vi "plot states.vi"(6 "Units":string(combo), 8 "Economizer?":bool, 9 "Power":dbl, 10 "fluid name":u16(ring)=17 items=["AIR.MIX", "AMARILLO.MIX", "EKOFISK.MIX", "GLFCOAST.MIX", "HIGHCO2.MIX", "HIGHN2.MIX", "NGSAMPLE.MIX", "R401A.MIX", "R401B.MIX", "R401C.MIX", "R402A.MIX", "R402B.MIX", "R403A.MIX", "R403B.MIX", "R405A.MIX", "R406A.MIX", "R407A.MIX", "R407B.MIX", "R407C.MIX", "R407D.MIX", "R407E.MIX", "R408A.MIX", "R409A.MIX", "R409B.MIX", "R410A.PPF", "R410B.MIX", "R411A.MIX", "R411B.MIX", "R412A.MIX", "R413A.MIX", "R414B.MIX", "R415A.MIX", "R415B.MIX", "R416A.MIX", "R417A.MIX", "R417B.MIX", "R417C.MIX", "R418A.MIX", "R419A.MIX", "R419B.MIX", "R420A.MIX", "R421A.MIX", "R421B.MIX", "R422A.MIX", "R422B.MIX", "R422C.MIX", "R422D.MIX", "R423A.MIX", "R424A.MIX", "R425A.MIX", "R426A.MIX", "R427A.MIX", "R428A.MIX", "R429A.MIX", "R430A.MIX", "R431A.MIX", "R432A.MIX", "R433A.MIX", "R433B.MIX", "R433C.MIX", "R434A.MIX", "R435A.MIX", "R436A.MIX", "R436B.MIX", "R437A.MIX", "R438A.MIX", "R439A.MIX", "R440A.MIX", "R441A.MIX", "R442A.MIX", "R443A.MIX", "R444A.MIX", "R444B.MIX", "R445A.MIX", "R446A.MIX", "R447A.MIX", "R448A.MIX", "R449A.MIX", "R449B.MIX", "R450A.MIX", "R451A.MIX", "R451B.MIX", "R452A.MIX", "R452B.MIX", "R452C.MIX", "R453A.MIX", "R454A.MIX", "R454B.MIX", "R454C.MIX", "R455A.MIX", "R456A.MIX", "R457A.MIX", "R459A.MIX", "R459B.MIX", "R460A.MIX", "R460B.MIX", "R500.MIX", "R501.MIX", "R502.MIX", "R503.MIX", "R504.MIX", "R507A.MIX", "R508A.MIX", "R508B.MIX", "R509A.MIX", "R510A.MIX", "R511A.MIX", "R512A.MIX", "R513A.MIX", "R513B.MIX", "R515A.MIX", "ammonia.fld", "butane.fld", "ethane.fld", "propane.fld", "R11.fld", "R113.fld", "R114.fld", "R115.fld", "R116.fld", "R12.fld", "R123.fld", "R124.fld", "R125.fld", "R13.fld", "R134a.fld", "R14.fld", "R141b.fld", "R142b.fld", "R143a.fld", "R152a.fld", "R161.fld", "R21.fld", "R218.fld", "R22.fld", "R227ea.fld", "R23.fld", "R236ea.fld", "R236fa.fld", "R245ca.fld", "R245fa.fld", "R32.fld", "R41.fld", "R1216.fld", "RC318.fld", "water.fld", "1butene.fld", "acetone.fld", "argon.fld", "benzene.fld", "c1cc6.fld", "c2butene.fld", "c3cc6.fld", "c4f10.fld", "c5f12.fld", "c11.fld", "c12.fld", "cf3i.fld", "CO.fld", "CO2.fld", "COS.fld", "cyclohex.fld", "cyclopen.fld", "cyclopro.fld", "D2.fld", "D2O.fld", "D4.fld", "D5.fld", "D6.fld", "decane.fld", "dee.fld", "dmc.fld", "dme.fld", "ebenzene.fld", "ethanol.fld", "ethylene.fld", "flourine.fld", "H2S.fld", "HCl.fld", "helium.fld", "heptane.fld", "hexane.fld", "hydrogen.fld", "ibutene.fld", "ihexane.fld", "ioctane.fld", "ipentane.fld", "isobutan.fld", "krypton.fld", "MD2M.fld", "MD3M.fld", "MD4M.fld", "MDM.fld", "methane.fld", "methanol.fld", "mlinolea.fld", "mlinolen.fld", "MM.fld", "moleate.fld", "mpalmita.fld", "mstearat.fld", "mxylene.fld", "N2O.fld", "neon.fld", "neopentn.fld", "NF3.fld", "nitrogen.fld", "nonane.fld", "novec649.fld", "octane.fld", "orthohyd.fld", "oxygen.fld", "parahyd.fld", "pentane.fld", "propylen.fld", "propyne.fld", "pxylene.fld", "R365MFC.fld", "R1233zd.fld", "R1234yf.fld", "R1234ze.fld", "RE143a.fld", "RE245cb2.fld", "RE245fa2.fld", "RE347mcc.fld", "sf6.fld", "SO2.fld", "T2butene.fld", "xenon.fld"], 11 "Data Cluster":T1) -> (0 "Ts output":cluster{dbl[], dbl[]}, 3 "ph output":cluster{dbl[], dbl[]})   [LabVIEW 2017]
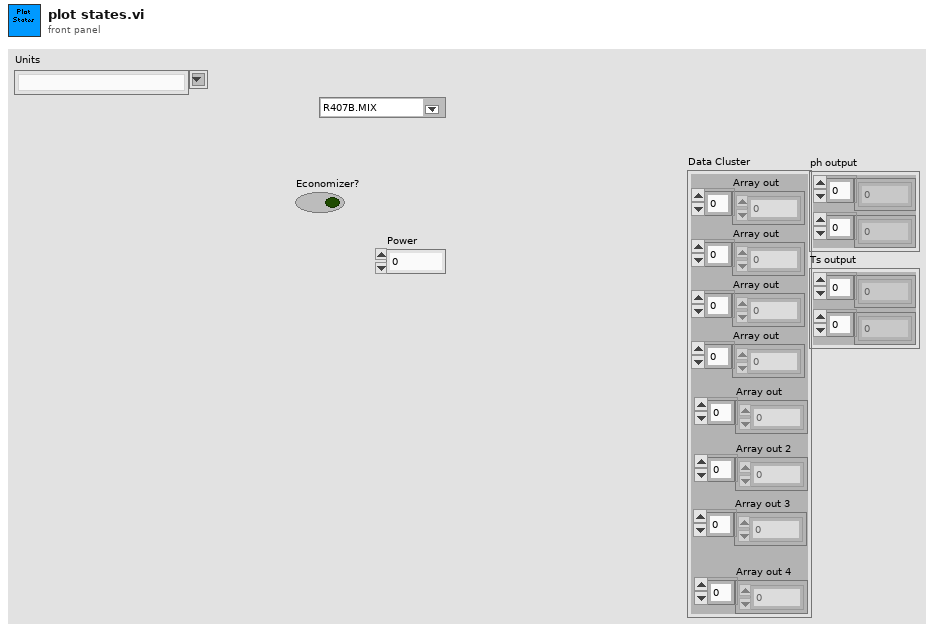
[diagram p1: front panel]
types:
  T1 = cluster{"Array out":dbl[], "Array out":dbl[], "Array out":dbl[], "Array out":dbl[], "Array out":dbl[], "Array out 2":dbl[], "Array out 3":dbl[], "Array out 4":dbl[]}
  T2 = enum16{"0", "PS", "HS", "T", "P", "TP", "TH", "TS", "PH", "PQ", "TQ"}
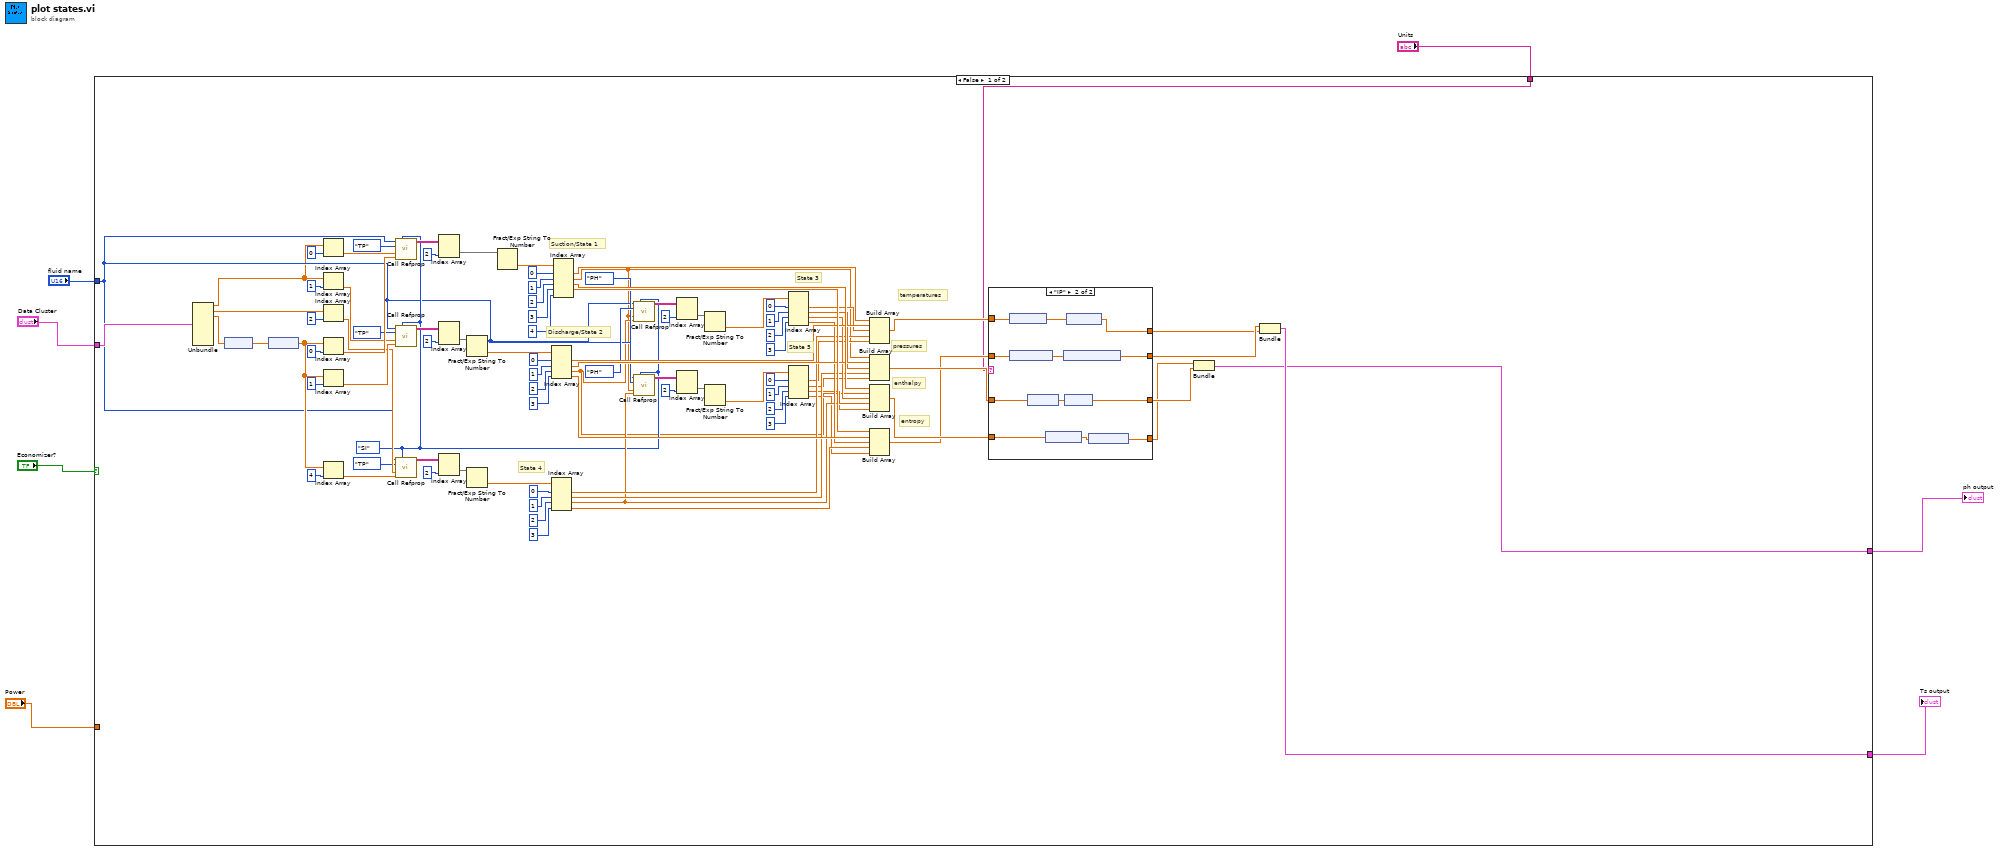
[diagram p0: block diagram]
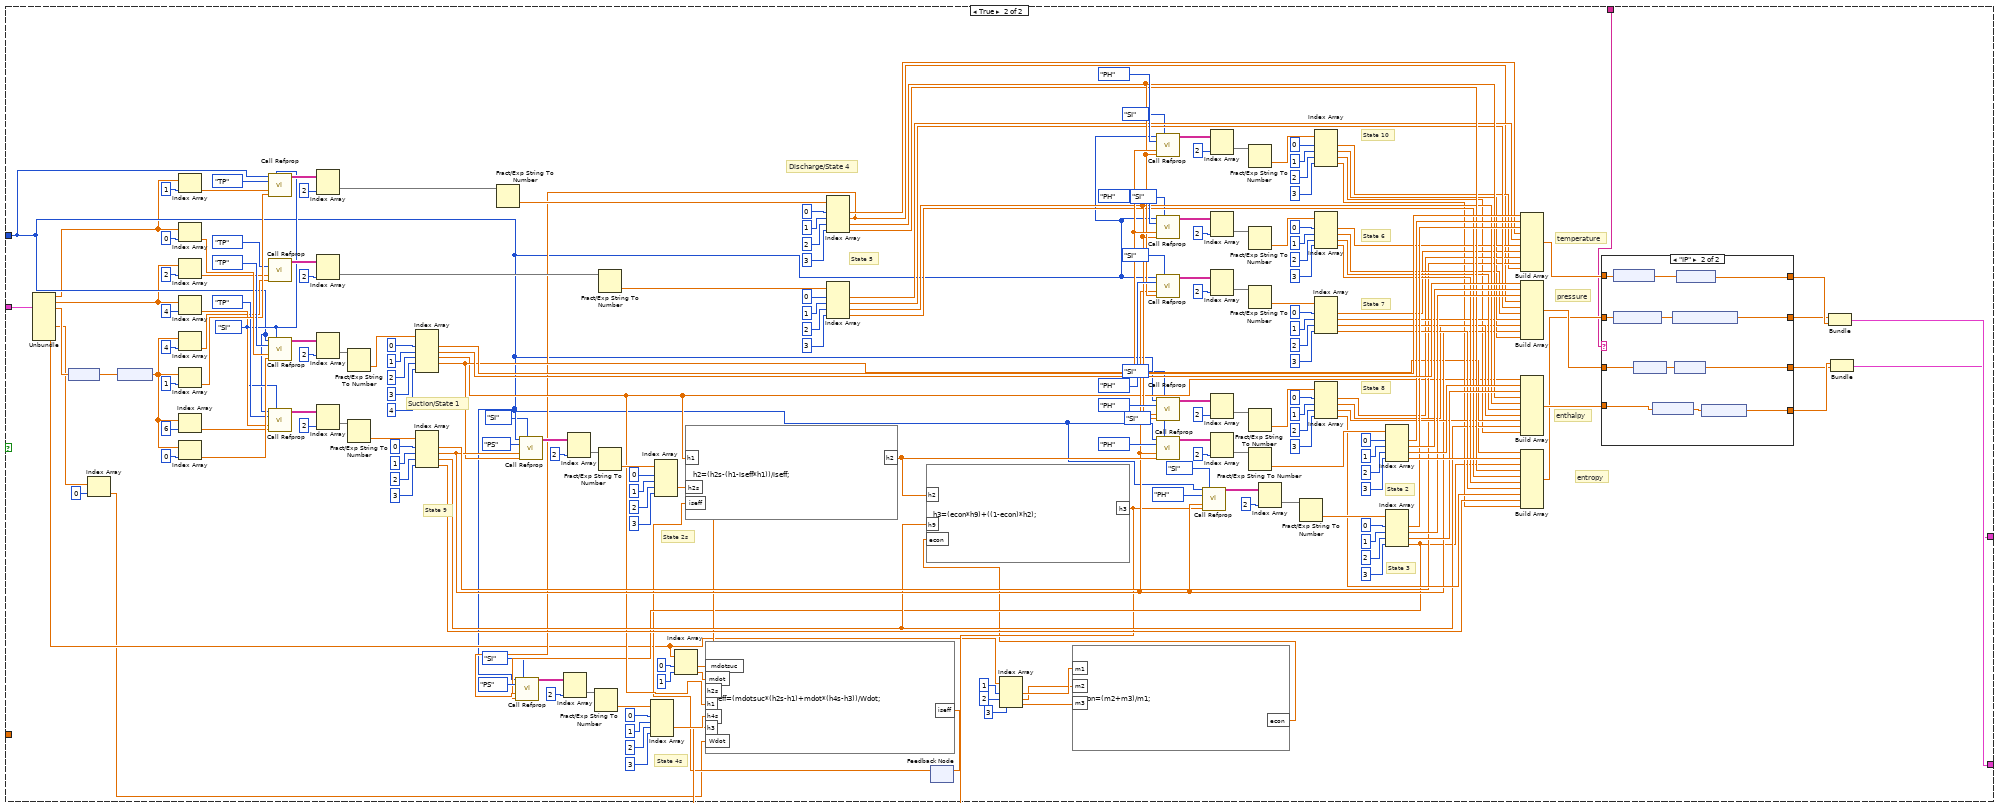
[diagram p3: hidden frame]
diagram:
  n1 = case shown="False" "Economizer?" {
    tunnel: [w24 w167] -> w6
    tunnel: [w23 w166] -> w5
    tunnel: "Data Cluster" -> [w22 w304]
    tunnel: "fluid name" -> [w21 w135]
    tunnel: "Power" -> [_ _]
    tunnel: "Units" -> [w10 w121]
    frame False {
      w25 = enum16{"SI", "IP"}."SI" ("units")
      # "State 5"
      # "State 4"
      # "State 3"
      # "Discharge/State 2"
      # "Suction/State 1"
      # "entropy"
      # "temperatures"
      # "enthalpy"
      # "pressures"
      n2 = Unbundle(w22) -> ("Array out"=w20:dbl[], "Array out"=w19:dbl[], "Array out"=w89:dbl[])  [unwired: 5 out]
      n3 = node(w89) -> (w90:dbl[unit][])
      n4 = node(w90) -> (w40:dbl[])
      n5 = Index Array(array=w20, index=0) -> (element=w101:dbl)
      n6 = Index Array(array=w20, index=1) -> (element=w83:dbl)
      n7 = Index Array(array=w19, index=2) -> (element=w54:dbl)
      n8 = Index Array(array=w40, index=0) -> (element=w100:dbl)
      n9 = Index Array(array=w40, index=1) -> (element=w82:dbl)
      n10 = Index Array(array=w40, index=4) -> (element=w53:dbl)
      n11 = call "Call Refprop.vi"("fluid name"=w21, "units"=w25, "InpCode"=T2."TP", "output_1"=w101, "output_2"=w100) -> ("data"=w99:string[][])  [unwired: 6 in, 4 out]
      n12 = call "Call Refprop.vi"("fluid name"=w21, "units"=w25, "InpCode"=T2."TP", "output_1"=w83, "output_2"=w82) -> ("data"=w81:string[][])  [unwired: 6 in, 4 out]
      n13 = call "Call Refprop.vi"("fluid name"=w21, "units"=w25, "InpCode"=T2."TP", "output_1"=w54, "output_2"=w53) -> ("data"=w52:string[][])  [unwired: 6 in, 4 out]
      n14 = Index Array(array=w99, index (col)=2 ("disabled index (col)")) -> (element=w97:string[])  [unwired: 1 in]
      n15 = Index Array(array=w81, index (col)=2 ("disabled index (col)")) -> (element=w79:string[])  [unwired: 1 in]
      n16 = Index Array(array=w52, index (col)=2 ("disabled index (col)")) -> (element=w50:string[])  [unwired: 1 in]
      n17 = Fract/Exp String To Number(string=w79) -> (number=w78:dbl[])  [unwired: 3 in, 1 out]
      n18 = Fract/Exp String To Number(string=w50) -> (number=w49:dbl[])  [unwired: 3 in, 1 out]
      n19 = Fract/Exp String To Number(string=w97) -> (number=w96:dbl[])  [unwired: 3 in, 1 out]
      n20 = Index Array(array=w78, index #1=0 ("index"), index #2=1 ("index"), index #3=2 ("index"), index #4=3 ("index")) -> (element #1=w72:dbl, element #2=w71:dbl, element #3=w9:dbl, element #4=w70:dbl)
      n21 = Index Array(array=w49, index #1=0 ("index"), index #2=1 ("index"), index #3=2 ("index"), index #4=3 ("index")) -> (element #1=w43:dbl, element #2=w42:dbl, element #3=w30:dbl, element #4=w41:dbl)
      n22 = Index Array(array=w96, index #1=0 ("index"), index #2=1 ("index"), index #3=2 ("index"), index #4=3 ("index"), index #5=4 ("index")) -> (element #1=w87:dbl, element #2=w8:dbl, element #3=w88:dbl, element #4=w86:dbl)  [unwired: 1 out]
      n23 = call "Call Refprop.vi"("fluid name"=w21, "units"=w25, "InpCode"=T2."PH", "output_1"=w8, "output_2"=w9) -> ("data"=w69:string[][])  [unwired: 6 in, 4 out]
      n24 = call "Call Refprop.vi"("fluid name"=w21, "units"=w25, "InpCode"=T2."PH", "output_1"=w8, "output_2"=w30) -> ("data"=w39:string[][])  [unwired: 6 in, 4 out]
      n25 = Index Array(array=w69, index (col)=2 ("disabled index (col)")) -> (element=w67:string[])  [unwired: 1 in]
      n26 = Index Array(array=w39, index (col)=2 ("disabled index (col)")) -> (element=w37:string[])  [unwired: 1 in]
      n27 = Fract/Exp String To Number(string=w67) -> (number=w66:dbl[])  [unwired: 3 in, 1 out]
      n28 = Fract/Exp String To Number(string=w37) -> (number=w36:dbl[])  [unwired: 3 in, 1 out]
      n29 = Index Array(array=w66, index #1=0 ("index"), index #2=1 ("index"), index #3=2 ("index"), index #4=3 ("index")) -> (element #1=w60:dbl, element #2=w59:dbl, element #3=w58:dbl, element #4=w57:dbl)
      n30 = Index Array(array=w36, index #1=0 ("index"), index #2=1 ("index"), index #3=2 ("index"), index #4=3 ("index")) -> (element #1=w29:dbl, element #2=w28:dbl, element #3=w27:dbl, element #4=w26:dbl)
      n31 = Build Array(w87, w72, w60, w43, w29) -> (w15:dbl[])
      n32 = Build Array(w8, w71, w59, w42, w28) -> (w18:dbl[])
      n33 = Build Array(w88, w9, w58, w30, w27) -> (w17:dbl[])
      n34 = Build Array(w86, w70, w57, w41, w26) -> (w16:dbl[])
      n35 = case shown="\"IP\"" w10 {
        tunnel: w18 -> [w107 w116]
        tunnel: w17 -> [w108 w115]
        tunnel: w16 -> [w106 w114]
        tunnel: w15 -> [w105 w113]
        tunnel: [w106 w112] -> w14
        tunnel: [w105 w111] -> w13
        tunnel: [w107 w110] -> w12
        tunnel: [w108 w109] -> w11
        frame "SI", Default {
        }
        frame "IP" {
          n36 = node(w113) -> (w118:dbl[unit][])
          n37 = node(w114) -> (w117:dbl[unit][])
          n38 = node(w116) -> (w119:dbl[unit][])
          n39 = node(w115) -> (w120:dbl[unit][])
          n40 = node(w117) -> (w112:dbl[])
          n41 = node(w119) -> (w110:dbl[])
          n42 = node(w118) -> (w111:dbl[])
          n43 = node(w120) -> (w109:dbl[])
        }
      }
      n44 = Bundle(w11, w12) -> (w23:cluster{dbl[], dbl[]})  [unwired: 1 in]
      n45 = Bundle(w14, w13) -> (w24:cluster{dbl[], dbl[]})  [unwired: 1 in]
    }
    frame True {
      w165 = enum16{"SI", "IP"}."SI" ("units")
      # "State 4s"
      # "entropy"
      # "temperature"
      # "enthalpy"
      # "pressure"
      # "State 2"
      # "State 10"
      # "State 8"
      # "State 7"
      # "State 6"
      # "State 5"
      # "State 2s"
      # "State 3"
      # "State 9"
      # "Discharge/State 4"
      # "Suction/State 1"
      n46 = Unbundle(w304) -> ("Array out"=w123:dbl[], "Array out"=w122:dbl[], "Array out"=w318:dbl[], "Array out"=w139:dbl[], "Array out 2"=w126:dbl[])  [unwired: 3 out]
      n47 = node(w318) -> (w319:dbl[unit][])
      n48 = Index Array(array=w126, index=0) -> (element=w125:dbl)
      n49 = node(w319) -> (w250:dbl[])
      n50 = Index Array(array=w123, index=1) -> (element=w314:dbl)
      n51 = Index Array(array=w123, index=0) -> (element=w330:dbl)
      n52 = Index Array(array=w122, index=2) -> (element=w269:dbl)
      n53 = Index Array(array=w122, index=4) -> (element=w300:dbl)
      n54 = Index Array(array=w250, index=4) -> (element=w268:dbl)
      n55 = Index Array(array=w250, index=1) -> (element=w313:dbl)
      n56 = Index Array(array=w250, index=6) -> (element=w299:dbl)
      n57 = Index Array(array=w250, index=0) -> (element=w329:dbl)
      n58 = call "Call Refprop.vi"("fluid name"=w135, "units"=w165, "InpCode"=T2."TP", "output_1"=w314, "output_2"=w313) -> ("data"=w312:string[][])  [unwired: 6 in, 4 out]
      n59 = call "Call Refprop.vi"("InpCode"=T2."TP", "output_1"=w269, "output_2"=w268) -> ("data"=w267:string[][])  [unwired: 8 in, 4 out]
      n60 = call "Call Refprop.vi"("fluid name"=w135, "units"=w165, "InpCode"=T2."TP", "output_1"=w330, "output_2"=w329) -> ("data"=w328:string[][])  [unwired: 6 in, 4 out]
      n61 = call "Call Refprop.vi"("fluid name"=w135, "units"=w165, "InpCode"=T2."TP", "output_1"=w300, "output_2"=w299) -> ("data"=w298:string[][])  [unwired: 6 in, 4 out]
      n62 = Index Array(array=w312, index (col)=2 ("disabled index (col)")) -> (element=w310:string[])  [unwired: 1 in]
      n63 = Index Array(array=w267, index (col)=2 ("disabled index (col)")) -> (element=w265:string[])  [unwired: 1 in]
      n64 = Index Array(array=w328, index (col)=2 ("disabled index (col)")) -> (element=w326:string[])  [unwired: 1 in]
      n65 = Index Array(array=w298, index (col)=2 ("disabled index (col)")) -> (element=w296:string[])  [unwired: 1 in]
      n66 = Fract/Exp String To Number(string=w326) -> (number=w325:dbl[])  [unwired: 3 in, 1 out]
      n67 = Fract/Exp String To Number(string=w296) -> (number=w295:dbl[])  [unwired: 3 in, 1 out]
      n68 = Index Array(array=w325, index #1=0 ("index"), index #2=1 ("index"), index #3=2 ("index"), index #4=3 ("index"), index #5=4 ("index")) -> (element #1=w212:dbl, element #2=w211:dbl, element #3=w159:dbl, element #4=w176:dbl)  [unwired: 1 out]
      n69 = Index Array(array=w295, index #1=0 ("index"), index #2=1 ("index"), index #3=2 ("index"), index #4=3 ("index")) -> (element #1=w184:dbl, element #2=w183:dbl, element #3=w182:dbl, element #4=w181:dbl)
      n70 = Fract/Exp String To Number(string=w310) -> (number=w309:dbl[])  [unwired: 3 in, 1 out]
      n71 = call "Call Refprop.vi"("fluid name"=w135, "units"=enum16{"SI", "IP"}."SI", "InpCode"=T2."PS", "output_1"=w183, "output_2"=w176) -> ("data"=w280:string[][])  [unwired: 6 in, 4 out]
      n72 = Index Array(array=w280, index (col)=2 ("disabled index (col)")) -> (element=w278:string[])  [unwired: 1 in]
      n73 = Fract/Exp String To Number(string=w265) -> (number=w264:dbl[])  [unwired: 3 in, 1 out]
      n74 = Fract/Exp String To Number(string=w278) -> (number=w277:dbl[])  [unwired: 3 in, 1 out]
      n75 = Index Array(array=w277, index #1=0 ("index"), index #2=1 ("index"), index #3=2 ("index"), index #4=3 ("index")) -> (element #3=w160:dbl)  [unwired: 3 out]
      n76 = Index Array(array=w139, index #1=0 ("index"), index #2=1 ("index")) -> (element #1=w162:dbl, element #2=w161:dbl)
      n77 = Index Array(array=w309, index #1=0 ("index"), index #2=1 ("index"), index #3=2 ("index"), index #4=3 ("index")) -> (element #1=w203:dbl, element #2=w149:dbl, element #3=w202:dbl, element #4=w201:dbl)
      n78 = Index Array(array=w264, index #1=0 ("index"), index #2=1 ("index"), index #3=2 ("index"), index #4=3 ("index")) -> (element #1=w200:dbl, element #2=w199:dbl, element #3=w198:dbl, element #4=w197:dbl)
      n79 = feedback #1() -> (w144:dbl)  [unwired: 1 in]
      n80 = formula code="h2=(h2s-(h1-iseff*h1))/iseff;"("h1"=w159, "h2s"=w160, "iseff"=w144) -> ("h2"=w213:dbl)
      n81 = Index Array(array=w139, index #1=1 ("index"), index #2=2 ("index"), index #3=3 ("index")) -> (element #1=w140:dbl, element #2=w138:dbl, element #3=w137:dbl)
      n82 = formula code="econ=(m2+m3)/m1;"("m2"=w138, "m3"=w137, "m1"=w140) -> ("econ"=w136:dbl)
      n83 = formula code="h3=(econ*h9)+((1-econ)*h2);"("h2"=w213, "h9"=w182, "econ"=w136) -> ("h3"=w146:dbl)
      n84 = call "Call Refprop.vi"("fluid name"=w135, "units"=enum16{"SI", "IP"}."SI", "InpCode"=T2."PH", "output_1"=w211, "output_2"=w202) -> ("data"=w230:string[][])  [unwired: 6 in, 4 out]
      n85 = call "Call Refprop.vi"("fluid name"=w135, "units"=enum16{"SI", "IP"}."SI", "InpCode"=T2."PH", "output_1"=w211, "output_2"=w198) -> ("data"=w258:string[][])  [unwired: 6 in, 4 out]
      n86 = call "Call Refprop.vi"("fluid name"=w135, "units"=enum16{"SI", "IP"}."SI", "InpCode"=T2."PH", "output_1"=w183, "output_2"=w202) -> ("data"=w248:string[][])  [unwired: 6 in, 4 out]
      n87 = call "Call Refprop.vi"("fluid name"=w135, "units"=enum16{"SI", "IP"}."SI", "InpCode"=T2."PH", "output_1"=w183, "output_2"=w198) -> ("data"=w239:string[][])  [unwired: 6 in, 4 out]
      n88 = call "Call Refprop.vi"("fluid name"=w135, "units"=enum16{"SI", "IP"}."SI", "InpCode"=T2."PH", "output_1"=w183, "output_2"=w213) -> ("data"=w221:string[][])  [unwired: 6 in, 4 out]
      n89 = call "Call Refprop.vi"("fluid name"=w135, "units"=enum16{"SI", "IP"}."SI", "InpCode"=T2."PH", "output_1"=w183, "output_2"=w146) -> ("data"=w289:string[][])  [unwired: 6 in, 4 out]
      n90 = Index Array(array=w230, index (col)=2 ("disabled index (col)")) -> (element=w228:string[])  [unwired: 1 in]
      n91 = Index Array(array=w258, index (col)=2 ("disabled index (col)")) -> (element=w256:string[])  [unwired: 1 in]
      n92 = Index Array(array=w248, index (col)=2 ("disabled index (col)")) -> (element=w246:string[])  [unwired: 1 in]
      n93 = Index Array(array=w239, index (col)=2 ("disabled index (col)")) -> (element=w237:string[])  [unwired: 1 in]
      n94 = Index Array(array=w221, index (col)=2 ("disabled index (col)")) -> (element=w219:string[])  [unwired: 1 in]
      n95 = Fract/Exp String To Number(string=w228) -> (number=w227:dbl[])  [unwired: 3 in, 1 out]
      n96 = Fract/Exp String To Number(string=w256) -> (number=w255:dbl[])  [unwired: 3 in, 1 out]
      n97 = Fract/Exp String To Number(string=w246) -> (number=w245:dbl[])  [unwired: 3 in, 1 out]
      n98 = Fract/Exp String To Number(string=w237) -> (number=w236:dbl[])  [unwired: 3 in, 1 out]
      n99 = Fract/Exp String To Number(string=w219) -> (number=w218:dbl[])  [unwired: 3 in, 1 out]
      n100 = Index Array(array=w289, index (col)=2 ("disabled index (col)")) -> (element=w287:string[])  [unwired: 1 in]
      n101 = Fract/Exp String To Number(string=w287) -> (number=w286:dbl[])  [unwired: 3 in, 1 out]
      n102 = Index Array(array=w227, index #1=0 ("index"), index #2=1 ("index"), index #3=2 ("index"), index #4=3 ("index")) -> (element #1=w180:dbl, element #2=w179:dbl, element #3=w178:dbl, element #4=w177:dbl)
      n103 = Index Array(array=w255, index #1=0 ("index"), index #2=1 ("index"), index #3=2 ("index"), index #4=3 ("index")) -> (element #1=w196:dbl, element #2=w195:dbl, element #3=w194:dbl, element #4=w193:dbl)
      n104 = Index Array(array=w245, index #1=0 ("index"), index #2=1 ("index"), index #3=2 ("index"), index #4=3 ("index")) -> (element #1=w192:dbl, element #2=w191:dbl, element #3=w190:dbl, element #4=w189:dbl)
      n105 = Index Array(array=w236, index #1=0 ("index"), index #2=1 ("index"), index #3=2 ("index"), index #4=3 ("index")) -> (element #1=w188:dbl, element #2=w187:dbl, element #3=w186:dbl, element #4=w185:dbl)
      n106 = Index Array(array=w218, index #1=0 ("index"), index #2=1 ("index"), index #3=2 ("index"), index #4=3 ("index")) -> (element #1=w210:dbl, element #2=w209:dbl, element #3=w208:dbl, element #4=w207:dbl)
      n107 = Index Array(array=w286, index #1=0 ("index"), index #2=1 ("index"), index #3=2 ("index"), index #4=3 ("index")) -> (element #1=w206:dbl, element #2=w205:dbl, element #3=w204:dbl, element #4=w148:dbl)
      n108 = call "Call Refprop.vi"("fluid name"=w135, "units"=enum16{"SI", "IP"}."SI", "InpCode"=T2."PS", "output_1"=w149, "output_2"=w148) -> ("data"=w157:string[][])  [unwired: 6 in, 4 out]
      n109 = Index Array(array=w157, index (col)=2 ("disabled index (col)")) -> (element=w155:string[])  [unwired: 1 in]
      n110 = Fract/Exp String To Number(string=w155) -> (number=w154:dbl[])  [unwired: 3 in, 1 out]
      n111 = Index Array(array=w154, index #1=0 ("index"), index #2=1 ("index"), index #3=2 ("index"), index #4=3 ("index")) -> (element #3=w147:dbl)  [unwired: 3 out]
      n112 = formula code="iseff=(mdotsuc*(h2s-h1)+mdot*(h4s-h3))/Wdot;"("mdotsuc"=w162, "mdot"=w161, "h2s"=w160, "h1"=w159, "h4s"=w147, "h3"=w146, "Wdot"=w125) -> ("iseff"=w145:dbl)
      n113 = feedback-in #1(w145) -> ()
      n114 = Build Array(w212, w210, w206, w203, w200, w196, w192, w188, w184, w180) -> (w171:dbl[])
      n115 = Build Array(w211, w209, w205, w149, w199, w195, w191, w187, w183, w179) -> (w173:dbl[])
      n116 = Build Array(w159, w208, w204, w202, w198, w194, w190, w186, w182, w178) -> (w175:dbl[])
      n117 = Build Array(w176, w207, w148, w201, w197, w193, w189, w185, w181, w177) -> (w169:dbl[])
      n118 = case shown="\"IP\"" w121 {
        tunnel: w175 -> [w334 w347]
        tunnel: [w334 w346] -> w174
        tunnel: w173 -> [w335 w345]
        tunnel: [w335 w344] -> w172
        tunnel: w171 -> [w337 w342]
        tunnel: [w337 w341] -> w170
        tunnel: w169 -> [w336 w339]
        tunnel: [w336 w338] -> w168
        frame "SI", Default {
        }
        frame "IP" {
          n119 = node(w342) -> (w343:dbl[unit][])
          n120 = node(w339) -> (w340:dbl[unit][])
          n121 = node(w345) -> (w348:dbl[unit][])
          n122 = node(w347) -> (w349:dbl[unit][])
          n123 = node(w340) -> (w338:dbl[])
          n124 = node(w348) -> (w344:dbl[])
          n125 = node(w343) -> (w341:dbl[])
          n126 = node(w349) -> (w346:dbl[])
        }
      }
      n127 = Bundle(w168, w170) -> (w167:cluster{dbl[], dbl[]})  [unwired: 1 in]
      n128 = Bundle(w174, w172) -> (w166:cluster{dbl[], dbl[]})  [unwired: 1 in]
    }
  }
  "Ts output" <- w6
  "ph output" <- w5
